vi "RT - Analyzing Turbine Data.vi"   [LabVIEW 2012]
uses:
  <vilib>/LabVIEW Targets/FPGA/cRIO/shared/nicrio_ModuleControls/nicrio_cRIO-9234_DataRatesRing2.ctl
  Type Defs/Command Datatype.ctl
  <vilib>/Platform/TimedLoop/XDataNode/timing_clust.ctl
  <vilib>/Platform/TimedLoop/XDataNode/nitl_modes.ctl
  <vilib>/Platform/TimedLoop/XDataNode/wakeup.ctl
  <vilib>/FPGAPlugInAG/cRIO-9074/niLvFpga_Open_cRIO-9074.vi
  <vilib>/FPGAPlugInAG/cRIO-9074/niLvFpga_Reset_cRIO-9074.vi
  <vilib>/Utility/error.llb/Error Cluster From Error Code.vi
  <vilib>/rvi/errors/niLvFpgaAdjustHostInterfaceError.vi
  <vilib>/FPGAPlugInAG/cRIO-9074/niLvFpga_Run_cRIO-9074.vi
  <vilib>/Analysis/2dsp.llb/Power Spectrum (DBL).vi
  <vilib>/FPGAPlugInAG/cRIO-9074/niLvFpga_Close_cRIO-9074.vi
  <vilib>/Platform/TimedLoop/XDataNode/XDataNode.xnode
  <vilib>/rvi/interface/nirviOpenFPGA/nirviOpenFPGA.xnode
  FPGA Bitfiles/FPGATarget_FPGA-SamplingTurbine_3297E995.lvbitx
  FPGA - Sampling Turbine.vi
  <vilib>/rvi/interface/nirviMethod/nirviMethod.xnode
  <vilib>/rvi/interface/nirviReadWriteControl/nirviReadWriteControl.xnode
  <vilib>/rvi/interface/nirviCloseFPGA/nirviCloseFPGA.xnode
  <vilib>/Platform/TimedLoop/XDataNode/XDNodeRunTimeDep.lvlib
  <vilib>/Analysis/NI_AALPro.lvlib
  <vilib>/FPGAPlugInAG/cRIO-9074/niLvFpga_ConfigureFifo_cRIO-9074.vi
  <vilib>/rvi/errors/niLvFpgaMergeErrorWithErrorCode.vi
  NiFpgaLv.dll
  <vilib>/FPGAPlugInAG/cRIO-9074/niLvFpga_ReadFifo_cRIO-9074.vi
panel:
  # "The real-time target application analyzes and scales the\ndata that is acquired and tranferred from the FPGA. It also communicates the turbine PWM attributes from the Windows target to the FPGA."
  # "NOTE: The real-time target front panel does not have\ncontrols/indicators as these should only be used for\ndebugging purposes as a deployed solution is headless."
types:
  T1 = typedef "Command Datatype.ctl" = cluster{"Cmd":string, "Data":variant}
  T2 = typedef "nicrio_cRIO-9234_DataRatesRing2.ctl" = u8
  T3 = typedef "XDNodeRunTimeDep.lvlib/timing_clust.ctl" = cluster{"Expected End [f-1]":u64, "Actual End [f-1]":u64, "Finished Late? [f-1]":bool, "Expected End [i-1]":u64, "Actual End [i-1]":u64, "Finished Late? [i-1]":bool, "Expected Start [i]":u64, "Actual Start [i]":u64, "Expected Start [f]":u64, "Actual Start [f]":u64, "Source Name":string, "Structure Name":string, "Period":i64, "Deadline":i64, "Offset":i64, "Start":i64, "Priority":i32, "Timeout":i32, "Mode":T4, "Wakeup Reason":T5, "Error":errorcluster, "Source Type":string, "Secondary Source Type":string, "Global End Time":u64, "Global Start Time":u64, "Frame Duration":u64, "Iteration Duration":u64, "Assigned CPU":i32, "I/O Scan Engine Mode":u32}
  T4 = typedef "XDNodeRunTimeDep.lvlib/nitl_modes.ctl" = enum32{"No Change", "Process missed periods, maintain original phase", "Discard missed periods, maintain original phase", "Process missed periods, ignore original phase", "Discard missed periods, ignore original phase"}
  T5 = typedef "XDNodeRunTimeDep.lvlib/wakeup.ctl" = enum32{"Normal", "Aborted", "Asynchronous wakeup", "Timing source error", "Timed loop error", "Timeout"}
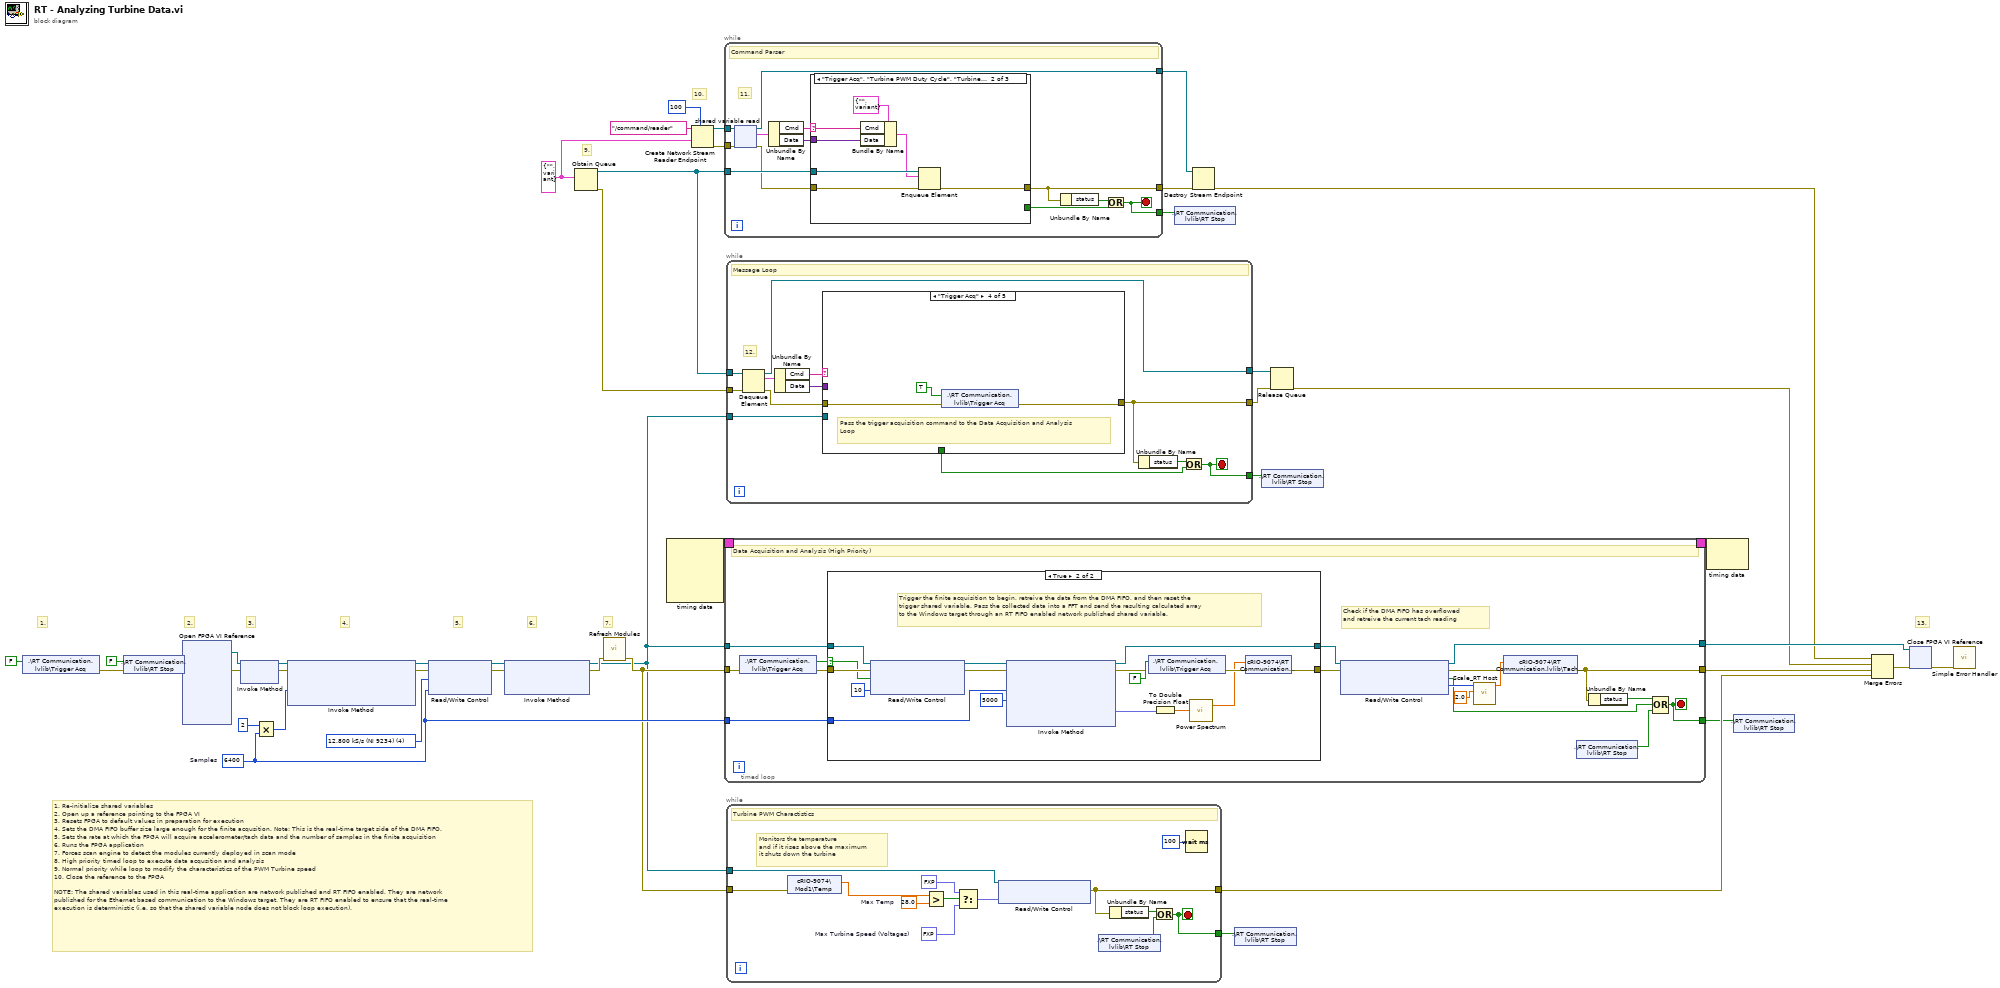
[diagram p0: block diagram]
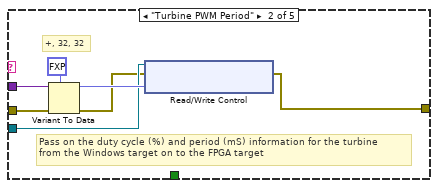
[diagram p3: hidden frame]
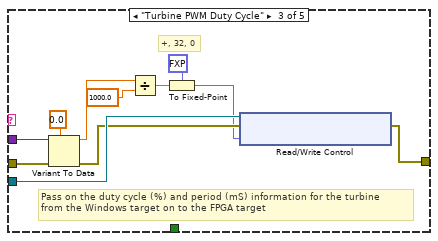
[diagram p4: hidden frame]
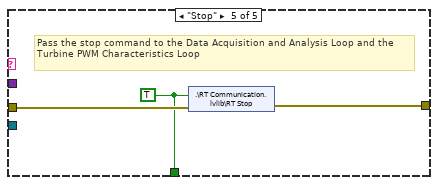
[diagram p5: hidden frame]
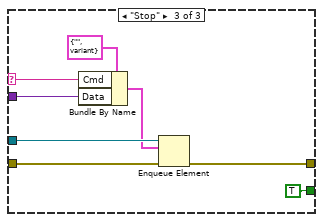
[diagram p7: hidden frame]
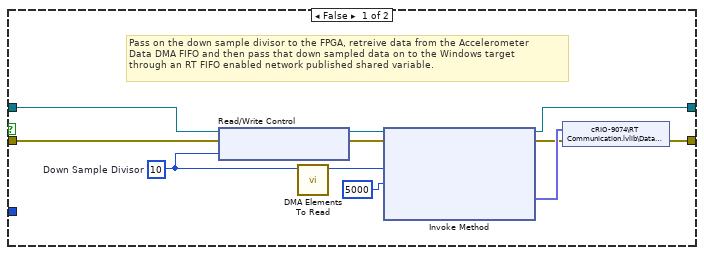
[diagram p8: hidden frame]
diagram:
  w12 = T1 {"Cmd"="", "Data"=variant}
  w32 = u32 6400  # Samples
  w40 = T2 4 items=["51.200 kS/s (NI 9234)"=1, "25.600 kS/s (NI 9234)"=2, "17.067 kS/s (NI 9234)"=3, "12.800 kS/s (NI 9234)"=4, "10.240 kS/s (NI 9234)"=5, "8.533 kS/s (NI 9234)"=6, "7.314 kS/s (NI 9234)"=7, "6.400 kS/s (NI 9234)"=8, "5.689 kS/s (NI 9234)"=9, "5.120 kS/s (NI 9234)"=10, "4.654 kS/s (NI 9234)"=11, "4.267 kS/s (NI 9234)"=12, "3.938 kS/s (NI 9234)"=13, "3.657 kS/s (NI 9234)"=14, "3.413 kS/s (NI 9234)"=15, "3.200 kS/s (NI 9234)"=16, "3.012 kS/s (NI 9234)"=17, "2.845 kS/s (NI 9234)"=18, "2.695 kS/s (NI 9234)"=19, "2.560 kS/s (NI 9234)"=20, "2.438 kS/s (NI 9234)"=21, "2.328 kS/s (NI 9234)"=22, "2.226 kS/s (NI 9234)"=23, "2.133 kS/s (NI 9234)"=24, "2.048 kS/s (NI 9234)"=25, "1.969 kS/s (NI 9234)"=26, "1.896 kS/s (NI 9234)"=27, "1.829 kS/s (NI 9234)"=28, "1.765 kS/s (NI 9234)"=29, "1.707 kS/s (NI 9234)"=30, "1.652 kS/s (NI 9234)"=31] ("Data Rate")
  # "10."
  # "9."
  # "13."
  # "7."
  # "6."
  # "5."
  # "4."
  # "3."
  # "2."
  # "1."
  # "1. Re-initialize shared variables \n2. Open up a reference pointing to the FPGA VI\n3. Resets FPGA to default values in preparation for execution \n4. Sets the DMA FIFO buffer size large enough for the finite acqusition. Note: This is the real-time target side of the DMA FIFO.\n5. Sets the rate at which the FPGA will acquire accelerometer/tach data and the number of samples in the finite acquisition\n6. Runs the FPGA application \n7. Forces scan engine to detect the modules currently deployed in scan mode\n8. High priority timed loop to execute data acqusition and analysis \n9. Normal priority while loop to modify the characteristics of the PWM Turbine speed\n10. Close the reference to the FPGA\n\nNOTE: The shared variables used in this real-time application are network published and RT FIFO enabled. They are network\npublished for the Ethernet based communication to the Windows target. They are RT FIFO enabled to ensure that the real-time\nexecution is deterministic (i.e. so that the shared variable node does not block loop execution)."
  n1 = shared-variable ".\\RT Communication.lvlib\\Trigger Acq"(FALSE ("Start")) -> (error out=w25:errorcluster)  [unwired: 1 in]
  n2 = shared-variable ".\\RT Communication.lvlib\\RT Stop"(FALSE ("Stop"), error in=w25) -> (error out=w27:errorcluster)
  n3 = xnode "Open FPGA VI Reference"("error in"=w27) -> ("FPGA VI Reference Out"=w42:refnum<k20>, "error out"=w41:errorcluster)  [unwired: 1 in]
  n4 = xnode "Invoke Method"("FPGA VI Reference In"=w42, "error in"=w41) -> ("FPGA VI Reference Out"=w38:refnum<k20>, "error out"=w35:errorcluster)
  n5 = Multiply(x=u32 2, y=w32) -> (x*y=w31:u32)
  n6 = xnode "Invoke Method"("FPGA VI Reference In"=w38, "error in"=w35, "Requested Depth"=w31) -> ("FPGA VI Reference Out"=w37:refnum<k20>, "error out"=w36:errorcluster)  [unwired: 1 out]
  n7 = xnode "Read/Write Control"("FPGA VI Reference In"=w37, "error in"=w36, "Data Rate"=w40, "Test Samples"=w32) -> ("FPGA VI Reference Out"=w39:refnum<k20>, "error out"=w23:errorcluster)
  n8 = xnode "Invoke Method"("FPGA VI Reference In"=w39, "error in"=w23) -> ("FPGA VI Reference Out"=w11:refnum<k20>, "error out"=w22:errorcluster)  [unwired: 1 in]
  n9 = Obtain Queue(element data type=w12) -> (queue out=w13:refnum<queue>, error out=w10:errorcluster)  [unwired: 4 in, 1 out]
  n10 = call <vilib>:"Refresh Modules.vi"("error in (no error)"=w22) -> ("error out"=w21:errorcluster)  [unwired: 10 in]
  n11 = node-c288() -> (w18:T3)  [unwired: 4 in]
  n12 = Create Network Stream Reader Endpoint(7:100 ("reader buffer size"), 9:w12, 11:"/command/reader" ("reader name")) -> (0:w14:errorcluster, 3:w15:refnum<k21>)  [unwired: 4 in]
  n13 = timed-loop {
    tunnel: [w60] -> w43
    tunnel: [w48] -> w30
    tunnel: w11 -> [w53]
    tunnel: w21 -> [w52]
    tunnel: w32 -> [w59]
    tunnel: [w45] -> w19
    timing: w18 -> [_]
    timing-out: [_] -> w17
    stop <- w45 stop-if-true
    # "Check if the DMA FIFO has overflowed\nand retreive the current tach reading"
    # "Data Acquisition and Analysis (High Priority)"
    n14 = shared-variable ".\\RT Communication.lvlib\\Trigger Acq"(error in=w52) -> (w54:bool, error out=w51:errorcluster)
    n15 = case shown="True" w54 {
      selector: w54 -> [_ w81]
      tunnel: w59 -> [_ w86]
      tunnel: w53 -> [w68 w85]
      tunnel: w51 -> [w67 w84]
      tunnel: [w71 w78] -> w58
      tunnel: [w63 w76] -> w57
      frame False {
        w62 = 10  # Down Sample Divisor
        # "Pass on the down sample divisor to the FPGA, retreive data from the Accelerometer\nData DMA FIFO and then pass that down sampled data on to the Windows target\nthrough an RT FIFO enabled network published shared variable."
        n16 = xnode "Read/Write Control"("FPGA VI Reference In"=w68, "error in"=w67, "Down Sample Divisor"=w62) -> ("FPGA VI Reference Out"=w66:refnum<k20>, "error out"=w65:errorcluster)
        n17 = call "DMA Elements To Read.vi"("Down Sample Divisor"=w62) -> ("Num of Elements"=w61:u32)  [unwired: 10 in]
        n18 = xnode "Invoke Method"("FPGA VI Reference In"=w66, "error in"=w65, "Number of Elements"=w61, "Timeout (ms)"=5000) -> ("FPGA VI Reference Out"=w71:refnum<k20>, "error out"=w64:errorcluster, "Data"=w70:fxp<+/-,24,4>[])  [unwired: 1 out]
        n19 = shared-variable "cRIO-9074\\RT Communication.lvlib\\Data Subset"(w70, error in=w64) -> (error out=w63:errorcluster)
      }
      frame True {
        # "Trigger the finite acquisition to begin, retreive the data from the DMA FIFO, and then reset the\ntrigger shared variable. Pass the collected data into a FFT and send the resulting calculated array\nto the Windows target through an RT FIFO enabled network published shared variable."
        n20 = xnode "Read/Write Control"("FPGA VI Reference In"=w85, "error in"=w84, "Start Test?"=w81, "Down Sample Divisor"=10) -> ("FPGA VI Reference Out"=w83:refnum<k20>, "error out"=w82:errorcluster)
        n21 = xnode "Invoke Method"("FPGA VI Reference In"=w83, "error in"=w82, "Number of Elements"=w86, "Timeout (ms)"=5000) -> ("FPGA VI Reference Out"=w78:refnum<k20>, "error out"=w79:errorcluster, "Data"=w73:fxp<+/-,24,4>[])  [unwired: 1 out]
        n22 = shared-variable ".\\RT Communication.lvlib\\Trigger Acq"(FALSE ("Start Ramp?"), error in=w79) -> (error out=w77:errorcluster)
        n23 = To Double Precision Float(number=w73) -> (double precision float=w72:dbl[])
        n24 = call-poly <vilib>:"Power Spectrum.vi"("X"=w72) -> ("Power Spectrum"=w74:dbl[])  [unwired: 1 out]
        n25 = shared-variable "cRIO-9074\\RT Communication.lvlib\\FFT"(w74, error in=w77) -> (error out=w76:errorcluster)
      }
    }
    n26 = xnode "Read/Write Control"("FPGA VI Reference In"=w58, "error in"=w57) -> ("FPGA VI Reference Out"=w60:refnum<k20>, "error out"=w49:errorcluster, "Overflow Occurred"=w47:bool, "Tach Period (uSec/pulse)"=w55:u32)
    n27 = call "Scale_RT Host.vi"("Number of Teeth in Sensor"=2.0, "Tach Period (uSec/pulse)"=w55) -> ("RPM"=w56:dbl)  [unwired: 9 in]
    n28 = shared-variable "cRIO-9074\\RT Communication.lvlib\\Tach RPMs"(w56, error in=w49) -> (error out=w48:errorcluster)
    n29 = shared-variable ".\\RT Communication.lvlib\\RT Stop"() -> (w50:bool)  [unwired: 1 in, 1 out]
    n30 = Unbundle By Name(w48) -> ("status"=w46:bool)
    n31 = Compound Arithmetic op=OR(w46, w47, w50) -> (w45:bool)
  }
  n32 = while {
    tunnel: w15 -> [w101]
    tunnel: w13 -> [w99]
    tunnel: w14 -> [w98]
    tunnel: [w94] -> w2
    tunnel: [w92] -> w4
    tunnel: [w91] -> w3
    stop <- w92 stop-if-true
    # "11."
    # "Command Parser"
    n33 = shared-variable-read(w101, w98) -> (w91:refnum<k21>, w97:errorcluster, w90:T1)  [unwired: 1 in, 1 out]
    n34 = Unbundle By Name(w90) -> ("Cmd"=w100:string, "Data"=w96:variant)
    n35 = case shown="\"Trigger Acq\", \"Turbine PWM Duty Cycle\", \"Turbine PWM Period\"" w100 {
      selector: w100 -> [_ w105 w112]
      tunnel: w99 -> [_ w108 w116]
      tunnel: w97 -> [w102 w109 w117]
      tunnel: w96 -> [_ w104 w111]
      tunnel: [w102 w107 w115] -> w94
      tunnel: [_ _ TRUE] -> w93
      frame Default {
      }
      frame "Trigger Acq", "Turbine PWM Duty Cycle", "Turbine PWM Period" {
        n36 = Bundle By Name(cluster=T1 {"Cmd"="", "Data"=variant}, "Cmd"=w105, "Data"=w104) -> (w103:T1)
        n37 = Enqueue Element(queue=w108, element=w103, error in (no error)=w109) -> (error out=w107:errorcluster)  [unwired: 1 in, 2 out]
      }
      frame "Stop" {
        n38 = Bundle By Name(cluster=T1 {"Cmd"="", "Data"=variant}, "Cmd"=w112, "Data"=w111) -> (w110:T1)
        n39 = Enqueue Element(queue=w116, element=w110, error in (no error)=w117) -> (error out=w115:errorcluster)  [unwired: 1 in, 2 out]
      }
    }
    n40 = Unbundle By Name(w94) -> ("status"=w95:bool)
    n41 = Or(x=w95, y=w93) -> (x .or. y?=w92:bool)
  }
  n42 = while {
    tunnel: w13 -> [w129]
    tunnel: w11 -> [w125]
    tunnel: w10 -> [w123]
    tunnel: [w121] -> w8
    tunnel: [w122] -> w9
    tunnel: [w118] -> w5
    stop <- w118 stop-if-true
    # "12."
    # "Message Loop"
    n43 = Dequeue Element(queue=w129, error in (no error)=w123) -> (queue out=w122:refnum<queue>, element=w128:T1, error out=w124:errorcluster)  [unwired: 1 in, 1 out]
    n44 = Unbundle By Name(w128) -> ("Cmd"=w127:string, "Data"=w126:variant)
    n45 = case shown="\"Trigger Acq\"" w127 {
      tunnel: w126 -> [_ w136 w147 _ _]
      tunnel: w125 -> [_ w134 w146 _ _]
      tunnel: w124 -> [w130 w133 w145 w151 w154]
      tunnel: [w130 w131 w138 w150 w153] -> w121
      tunnel: [_ _ _ _ w152] -> w119
      frame Default {
      }
      frame "Turbine PWM Period" {
        # "Pass on the duty cycle (%) and period (mS) information for the turbine\nfrom the Windows target on to the FPGA target"
        # "+, 32, 32"
        n46 = Variant To Data(error in=w133, type=fxp<+,32,32> 0.0, Variant=w136) -> (data=w135:fxp<+,32,32>, error out=w132:errorcluster)
        n47 = xnode "Read/Write Control"("FPGA VI Reference In"=w134, "error in"=w132, "Turbine PWM Period"=w135) -> ("error out"=w131:errorcluster)  [unwired: 1 out]
      }
      frame "Turbine PWM Duty Cycle" {
        # "Pass on the duty cycle (%) and period (mS) information for the turbine\nfrom the Windows target on to the FPGA target"
        # "+, 32, 0"
        n48 = Variant To Data(error in=w145, type=0.0, Variant=w147) -> (data=w143:dbl, error out=w144:errorcluster)
        n49 = Divide(x=w143, y=1000.0) -> (x/y=w141:dbl)
        n50 = To Fixed-Point(fixed-point type=fxp<+/-,32,0> 0.0, number=w141) -> (fixed-point=w139:fxp<+/-,32,0>)
        n51 = xnode "Read/Write Control"("FPGA VI Reference In"=w146, "error in"=w144, "Turbine PWM Duty Cycle"=w139) -> ("error out"=w138:errorcluster)  [unwired: 1 out]
      }
      frame "Trigger Acq" {
        # "Pass the trigger acquisition command to the Data Acquisition and Analysis Loop"
        n52 = shared-variable ".\\RT Communication.lvlib\\Trigger Acq"(TRUE, error in=w151) -> (error out=w150:errorcluster)
      }
      frame "Stop" {
        w152 = TRUE
        # "Pass the stop command to the Data Acquisition and Analysis Loop and the Turbine PWM Characteristics Loop"
        n53 = shared-variable ".\\RT Communication.lvlib\\RT Stop"(w152, error in=w154) -> (error out=w153:errorcluster)
      }
    }
    n54 = Unbundle By Name(w121) -> ("status"=w120:bool)
    n55 = Or(x=w120, y=w119) -> (x .or. y?=w118:bool)
  }
  n56 = while {
    tunnel: w11 -> [w163]
    tunnel: [w166] -> w34
    tunnel: w21 -> [w161]
    tunnel: [w164] -> w20
    stop <- w164 stop-if-true
    w159 = 28.0  # Max Temp
    w157 = fxp<+/-,20,5> 8.0  # Max Turbine Speed (Voltages)
    # "Monitors the temperature\nand if it rises above the maximum\nit shuts down the turbine"
    # "Turbine PWM Charactistics"
    n57 = shared-variable "cRIO-9074\\Mod1\\Temp"(error in=w161) -> (w160:dbl)  [unwired: 1 out]
    n58 = Greater?(x=w160, y=w159) -> (0:w158:bool)
    n59 = Select(t=fxp<+/-,20,5> 0.0, s=w158, f=w157) -> (s? t:f=w155:fxp<+/-,20,5>)
    n60 = xnode "Read/Write Control"("FPGA VI Reference In"=w163, "Turbine Max Voltage"=w155) -> ("error out"=w166:errorcluster)  [unwired: 1 in, 1 out]
    n61 = shared-variable ".\\RT Communication.lvlib\\RT Stop"() -> (w165:bool)  [unwired: 1 in, 1 out]
    n62 = Unbundle By Name(w166) -> ("status"=w167:bool)
    n63 = Or(x=w167, y=w165) -> (x .or. y?=w164:bool)
    n64 = Wait (ms)(milliseconds to wait=u32 100) -> ()  [unwired: 1 out]
  }
  n65 = shared-variable ".\\RT Communication.lvlib\\RT Stop"(w4) -> ()  [unwired: 1 in, 1 out]
  n66 = Destroy Stream Endpoint(8:w2, 11:w3) -> (0:w1:errorcluster)
  n67 = shared-variable ".\\RT Communication.lvlib\\RT Stop"(w20) -> ()  [unwired: 1 in, 1 out]
  n68 = shared-variable ".\\RT Communication.lvlib\\RT Stop"(w5) -> ()  [unwired: 1 in, 1 out]
  n69 = Release Queue(queue=w9, error in (no error)=w8) -> (error out=w6:errorcluster)  [unwired: 1 in, 2 out]
  n70 = node-c288(w17) -> ()  [unwired: 1 out]
  n71 = shared-variable ".\\RT Communication.lvlib\\RT Stop"(w19) -> ()  [unwired: 1 in, 1 out]
  n72 = Merge Errors(w1, w6, w30, w34) -> (w29:errorcluster)
  n73 = xnode "Close FPGA VI Reference"("FPGA VI Reference In"=w43, "error in"=w29) -> ("error out"=w28:errorcluster)
  n74 = call <vilib>:"Simple Error Handler.vi"("error in (no error)"=w28) -> ()  [unwired: 4 in, 5 out]
